vi "sqlite test.vi"() -> ()   [LabVIEW 2013, in "Medimatic.lvlib"]
uses:
  Medimatic.lvlib
  <userlib>/LVT/SQLite/Core/Insert/SQLite_Insert Row.vi
  <userlib>/LVT/SQLite/Core/Tables/SQLite_Drop Table.vi
  <userlib>/LVT/SQLite/Core/Tables/SQLite_Clear Table.vi
  <userlib>/LVT/SQLite/Core/Update/SQLite_Update Multiple.vi
  <userlib>/LVT/SQLite/Core/Update/SQLite_Update Single.vi
  <userlib>/LVT/SQLite/Core/Tables/SQLite_List Columns.vi
  <userlib>/LVT/SQLite/Core/Tables/SQLite_Create Table.vi
panel:
  out "Columns":string[](array[string])
  out "All Results Before Delete":string[][](array[string])
  out "DB OK?":bool
  out "Results":string[][](array[string])
  in  "DB Path":string="c:\\test.3db"
  in  "Tabe Name":string="TestTable"
  in  "Columns 2":string[](array[string])=["PassFail", "Value"]
  in  "error in (no error)":errorcluster
  out "error out":errorcluster
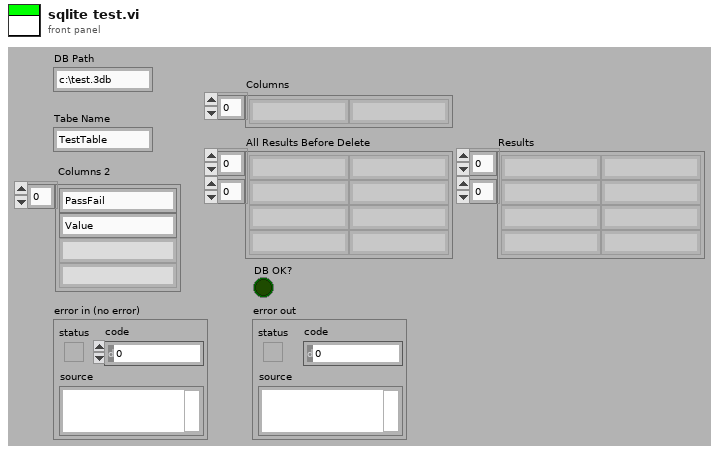
[diagram p1: front panel]
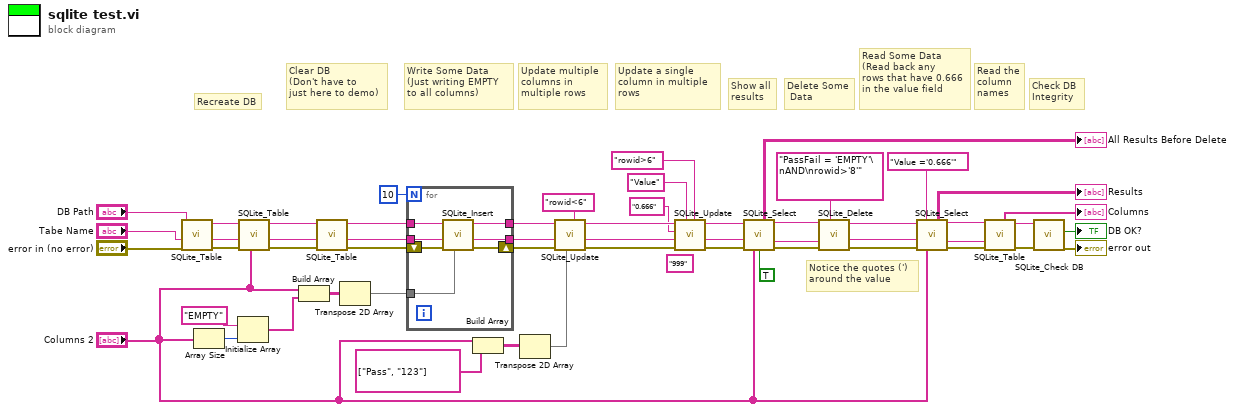
[diagram p0: block diagram]
diagram:
  (unwired) "999" ("Value")
  # "Read the\ncolumn\nnames"
  # "Show all\nresults"
  # "Delete Some\n Data"
  # "Check DB\nIntegrity"
  # "Notice the quotes (')\naround the value"
  # "Read Some Data\n(Read back any\nrows that have 0.666\nin the value field"
  # "Update a single\ncolumn in multiple\nrows"
  # "Update multiple\ncolumns in\nmultiple rows"
  # "Write Some Data\n(Just writing EMPTY\nto all columns)"
  # "Clear DB\n(Don't have to\njust here to demo)"
  # "Recreate DB"
  n1 = call-poly <userlib>:"SQLite_Table.vi"("DB Path"="DB Path", "Table Name"="Tabe Name", "error in (no error)"="error in (no error)") -> ("DB Path Out"=w40:string, "Table Name Out"=w38:string, "error out"=w39:errorcluster)  [unwired: 5 in]
  n2 = Array Size(array="Columns 2") -> (size(s)=w34:i32)
  n3 = Initialize Array("EMPTY" ("element"), w34) -> (w35:string[])
  n4 = call-poly <userlib>:"SQLite_Table.vi"("DB Path"=w40, "Table Name"=w38, "error in (no error)"=w39, "Columns"="Columns 2") -> ("DB Path Out"=w41:string, "Table Name Out"=w37:string, "error out"=w36:errorcluster)  [unwired: 4 in]
  n5 = Build Array("Columns 2", w35) -> (w3:string[][])
  n6 = call-poly <userlib>:"SQLite_Table.vi"("DB Path"=w41, "Table Name"=w37, "error in (no error)"=w36) -> ("DB Path Out"=w42:string, "Table Name Out"=w1:string, "error out"=w8:errorcluster)  [unwired: 5 in]
  n7 = Transpose 2D Array(2D array=w3) -> (transposed array=w2:string[][])
  n8 = for {
    N: 10 -> [_]
    tunnel: w42 -> [w61]
    tunnel: w1 -> [w60]
    tunnel: [w57] -> w48
    tunnel: [w56] -> w47
    tunnel: w2 -> [w55]
    shift-right: [w58] -> w7
    shift-left: w8 -> [w59]
    n9 = call-poly <userlib>:"SQLite_Insert.vi"("Column/Value Pairs"=w55, "error in"=w59, "Table Name"=w60, "DB Path"=w61) -> ("error out"=w58:errorcluster, "Tabe Name Out"=w56:string, "DB Path Out"=w57:string)  [unwired: 3 in]
  }
  n10 = Build Array("Columns 2", string[] ["Pass", "123"] ("Field Value Pairs")) -> (w44:string[][])
  n11 = Transpose 2D Array(2D array=w44) -> (transposed array=w43:string[][])
  n12 = call-poly <userlib>:"SQLite_Update.vi"("Where clause"="rowid<6", "Column/Value Pairs"=w43, "error in (no error)"=w7, "Tabe Name"=w47, "DB Path"=w48) -> ("error out"=w51:errorcluster, "Tabe NameOut"=w49:string, "DB Path Out"=w50:string)  [unwired: 2 in]
  n13 = call-poly <userlib>:"SQLite_Update.vi"("Where clause"="rowid>6", "Column"="Value" ("Field"), "error in"=w51, "Tabe Name"=w49, "Value"="0.666", "DB Path"=w50) -> ("error out"=w20:errorcluster, "Tabe NameOut"=w5:string, "DB Path Out"=w18:string)  [unwired: 1 in]
  n14 = call <userlib>:"SQLite_Select.vi"("DB Path"=w18, "Table Name"=w5, "error in (no error)"=w20, "Columns"="Columns 2", "Distinct"=TRUE) -> ("Results"=→"All Results Before Delete":string[][], "DB Path Out"=w17:string, "Table Name Out"=w6:string, "error out"=w19:errorcluster)  [unwired: 7 in]
  n15 = call <userlib>:"SQLite_Delete.vi"("Where Clause"="PassFail = 'EMPTY'\nAND\nrowid>'8'", "error in (no error)"=w19, "Table Name"=w6, "DB Path"=w17) -> ("error out"=w24:errorcluster, "Table Name Out"=w23:string, "DB Path Out"=w22:string)  [unwired: 3 in]
  n16 = call <userlib>:"SQLite_Select.vi"("DB Path"=w22, "Where Clause"="Value ='0.666'", "Table Name"=w23, "error in (no error)"=w24, "Columns"="Columns 2") -> ("Results"=→"Results":string[][], "DB Path Out"=w13:string, "Table Name Out"=w11:string, "error out"=w14:errorcluster)  [unwired: 7 in]
  n17 = call-poly <userlib>:"SQLite_Table.vi"("DB Path"=w13, "Table Name"=w11, "error in (no error)"=w14) -> ("Columns"=→"Columns":string[], "DB Path Out"=w10:string, "error out"=w15:errorcluster)  [unwired: 4 in, 1 out]
  n18 = call <userlib>:"SQLite_Check DB.vi"("error in (no error)"=w15, "DB Path"=w10) -> ("error out"=→"error out":errorcluster, "OK?"=→"DB OK?":bool)  [unwired: 7 in, 1 out]
